vi "ROI overlay test.vi"() -> ()   [LabVIEW 2013]
panel:
  out "ms between image":u32
  out "Frame Rate":dbl
  in  "Stop (F)":bool
  out "Image Out":T1(plugin-control)
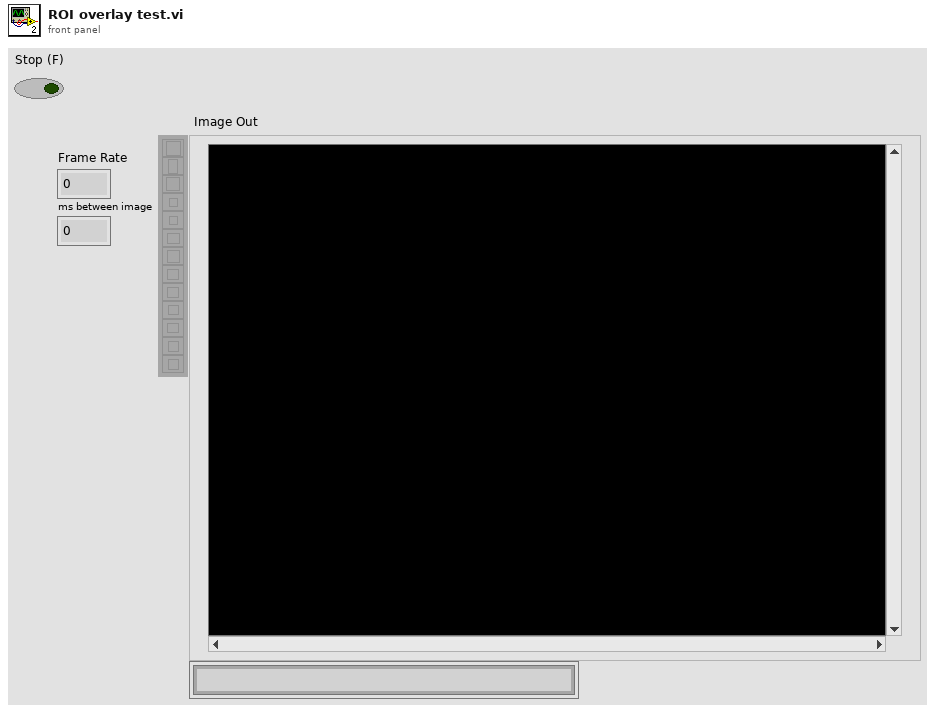
[diagram p1: front panel]
types:
  T1 = typedef "IMAQ Image.ctl" = refnum<image>
  T2 = typedef "ROI Descriptor" = cluster{"Global Rectangle":i32[], "Contours":cluster{"ID":enum32{"External", "Internal"}, "Type":u32, "Coordinates":i32[]}[]}
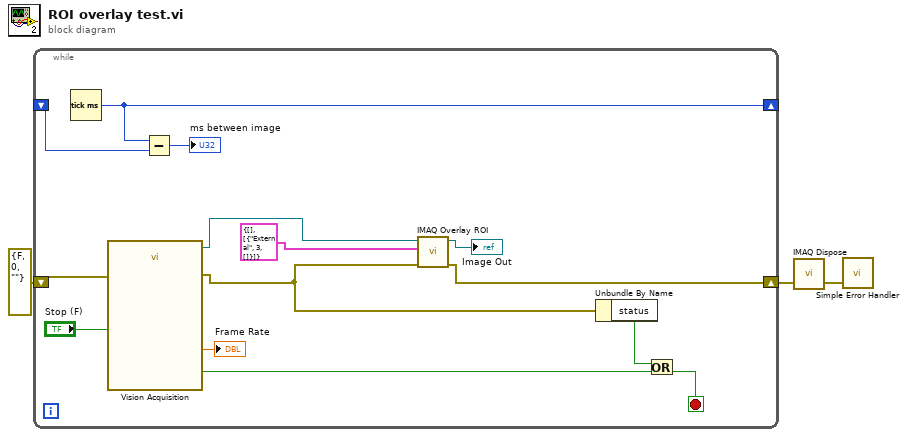
[diagram p0: block diagram]
diagram:
  n1 = while {
    shift-right: [w14] -> _
    shift-left: _ -> [w13]
    shift-right: [w4] -> w3
    shift-left: errorcluster {"status"=FALSE, "code"=0, "source"=""} ("error out") -> [w10]
    stop <- w11 stop-if-true
    n2 = Tick Count (ms)() -> (millisecond timer value=w14:u32)
    n3 = call "Vision Acquisition"("Stop (F)"="Stop (F)", "error in"=w10) -> ("Image Out"=w7:T1, "Frame Rate"=→"Frame Rate":dbl, "Stopped"=w16:bool, "error out"=w5:errorcluster)  [unwired: 22 in]
    n4 = Subtract(x=w14, y=w13) -> (x-y=→"ms between image":u32)
    n5 = call "IMAQ Overlay ROI"("error in (no error)"=w5, "ROI Descriptor"=T2 {"Global Rectangle"=[], "Contours"=[{"ID"=enum."External", "Type"=3, "Coordinates"=[]}]}, "Image"=w7) -> ("error out"=w4:errorcluster, "Image Out"=→"Image Out":T1)  [unwired: 7 in]
    n6 = Unbundle By Name(w5) -> ("status"=w9:bool)
    n7 = Or(x=w9, y=w16) -> (x .or. y?=w11:bool)
  }
  n8 = call "IMAQ Dispose"("error in (no error)"=w3) -> ("error out"=w1:errorcluster)  [unwired: 5 in]
  n9 = call <vilib>:"Simple Error Handler.vi"("error in (no error)"=w1) -> ()  [unwired: 4 in, 5 out]
